vi "GetMDT69Value.vi"(8 "error in (no error)":errorcluster, 10 "Channel":string, 11 "VISA resource name":refnum<visa-resource-name>) -> (0 "error out":errorcluster, 2 "Value":string, 3 "VISA resource name":refnum<visa-resource-name>)   [LabVIEW 2020]
uses:
  <userlib>/_MGI/Error Handling/MGI Suppress Error Code/MGI Suppress Error Code (Scalar).vi
  <userlib>/_MGI/Error Handling/MGI Suppress Error Code/MGI Suppress Error Code (Array).vi
  <vilib>/regexp/Match Regular Expression.xnode
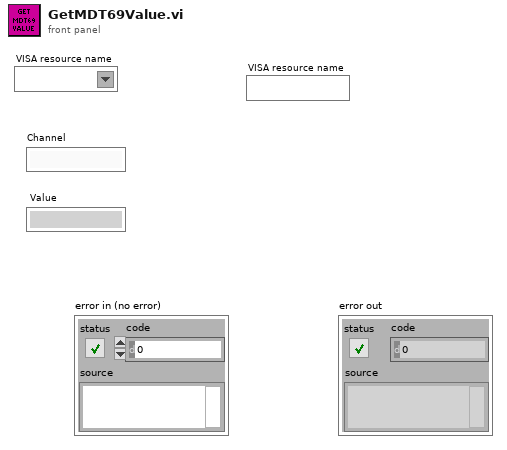
[diagram p1: front panel]
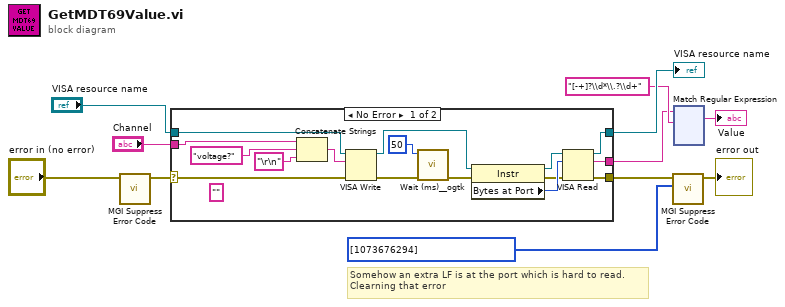
[diagram p0: block diagram]
diagram:
  # "Somehow an extra LF is at the port which is hard to read.\nClearning that error"
  n1 = call-poly <userlib>:"MGI Suppress Error Code.vi"("Error In"="error in (no error)") -> ("Error Out"=w4:errorcluster)  [unwired: 5 in, 1 out]
  n2 = case shown="No Error" w4 {
    selector: w4 -> [w23 w29]
    tunnel: [w12 w29] -> w3
    tunnel: "VISA resource name" -> [w24 w28]
    tunnel: [w15 w28] -> w10
    tunnel: "Channel" -> [w27 _]
    tunnel: [w19 _] -> w6
    frame No Error {
      (unwired) ""
      n3 = Concatenate Strings(w27, "voltage?" ("string"), "\r\n" ("string")) -> (w25:string)
      n4 = VISA Write(VISA resource name=w24, write buffer=w25, error in (no error)=w23) -> (VISA resource name out=w18:refnum<visa-resource-name>, error out=w21:errorcluster)  [unwired: 1 out]
      n5 = call <userlib>:"Wait (ms)__ogtk.vi"("error in (no error)"=w21, "milliseconds to wait"=u32 50) -> ("error out"=w14:errorcluster)  [unwired: 8 in, 1 out]
      n6 = property class="Instr"(reference=w18, error in=w14) -> (reference out=w17:refnum<visa-resource-name>, error out=w13:errorcluster, "Bytes at Port"=w16:u32)
      n7 = VISA Read(VISA resource name=w17, byte count=w16, error in (no error)=w13) -> (VISA resource name out=w15:refnum<visa-resource-name>, read buffer=w19:string, error out=w12:errorcluster)  [unwired: 1 out]
    }
    frame Error {
    }
  }
  "VISA resource name" <- w10
  n8 = call-poly <userlib>:"MGI Suppress Error Code.vi"("Error Codes[]"=i32[] [1073676294] ("Error Codes to Filter"), "Error In"=w3) -> ("Error Out"=→"error out":errorcluster)  [unwired: 4 in, 1 out]
  n9 = xnode "Match Regular Expression"("input string"=w6, "regular expression"="[-+]?\\d*\\.?\\d+") -> ("whole match"=→"Value":string)  [unwired: 4 in, 4 out]
